vi "Weighted_Cross_Moments_1.vi"(0 "Cluster 1":T2={"Colour"=0, "Inst type"=enum."Pitot-static tube", "Inst name"="Manometer voltage", "Symbol"="U", "Code name"="", "Extra Info"="U", "Inst Array"=enum."PWA", "Index"=0, "Voltage Index"=0, "Extra Titles"=[], "Extra Values"=[], "Eng Values"=[], "Time (ms)"=[], "TT / Voltage"=[], "U"=0.0, "u^2"=0.0, "u^3"=0.0, "u^4"=0.0, "Skew_u"=0.0, "Kurt_u"=0.0, "Sd Error in Mean"=0.0, "% u'/U"=0.0, "X"=0.0, "Y"=0.0, "Z"=0.0, "Spectra"={"First Name"="", "Second Name"="", "X axis name"="", "Y axis name"="", "X array"=[], "Y array"=[]}, "Autocorrelation"={"First Name"="", "Second Name"="", "X axis name"="", "Y axis name"="", "X array"=[], "Y array"=[]}, "Timescale integral to 25%"=0.0, "Sd Error in Variance"=0.0, "Calib File"=path "", "Calib Constants"=[], "Histogram"={"First Name"="", "Second Name"="", "X axis name"="", "Y axis name"="", "X array"=[], "Y array"=[]}, "Output Position"=FALSE, "Full Stats"=FALSE} {"Sd Error in Variance" format="%.2f"; "Skew_u" format="%.2f"; "% u'/U" format="%.2f"; "Sd Error in Mean" format="%.2f"; "Kurt_u" format="%.2f"; "u^4" format="%.2f"; "u^3" format="%.2f"; "U" format="%.2f"; "u^2" format="%.2f"}, 1 "Cluster 2":T2={"Colour"=0, "Inst type"=enum."Pitot-static tube", "Inst name"="Manometer voltage", "Symbol"="U", "Code name"="", "Extra Info"="U", "Inst Array"=enum."PWA", "Index"=0, "Voltage Index"=0, "Extra Titles"=[], "Extra Values"=[], "Eng Values"=[], "Time (ms)"=[], "TT / Voltage"=[], "U"=0.0, "u^2"=0.0, "u^3"=0.0, "u^4"=0.0, "Skew_u"=0.0, "Kurt_u"=0.0, "Sd Error in Mean"=0.0, "% u'/U"=0.0, "X"=0.0, "Y"=0.0, "Z"=0.0, "Spectra"={"First Name"="", "Second Name"="", "X axis name"="", "Y axis name"="", "X array"=[], "Y array"=[]}, "Autocorrelation"={"First Name"="", "Second Name"="", "X axis name"="", "Y axis name"="", "X array"=[], "Y array"=[]}, "Timescale integral to 25%"=0.0, "Sd Error in Variance"=0.0, "Calib File"=path "", "Calib Constants"=[], "Histogram"={"First Name"="", "Second Name"="", "X axis name"="", "Y axis name"="", "X array"=[], "Y array"=[]}, "Output Position"=FALSE, "Full Stats"=FALSE} {"Sd Error in Variance" format="%.2f"; "Skew_u" format="%.2f"; "% u'/U" format="%.2f"; "Sd Error in Mean" format="%.2f"; "Kurt_u" format="%.2f"; "u^4" format="%.2f"; "u^3" format="%.2f"; "U" format="%.2f"; "u^2" format="%.2f"}, 5 "Shift in":dbl[](array[numeric]) format="%.2f") -> (17 "output cluster":T1 {"u^2w^2" format="%.2f"; "u^3w" format="%.2f"; "uw^3" format="%.2f"; "uw/u'w'" format="%.2f"; "uw^2" format="%.2f"; "u^2w" format="%.2f"; "uw" format="%.2f"}, 19 "Shift out":dbl[](array[numeric]) format="%.2f")   [LabVIEW 2011]
uses:
  Controls/Analysis_info_cluster.ctl
  Controls/Inst_type.ctl
  Controls/Instrument_Array.ctl
  Controls/XY_Plot_Cluster.ctl
  Controls/Correlation_cluster1.ctl
  Globals/Meas_global.vi
panel:
  in  "interp. method":i32(ring) items=["nearest", "linear", "spline", "cubic Hermite", "Lagrange"]
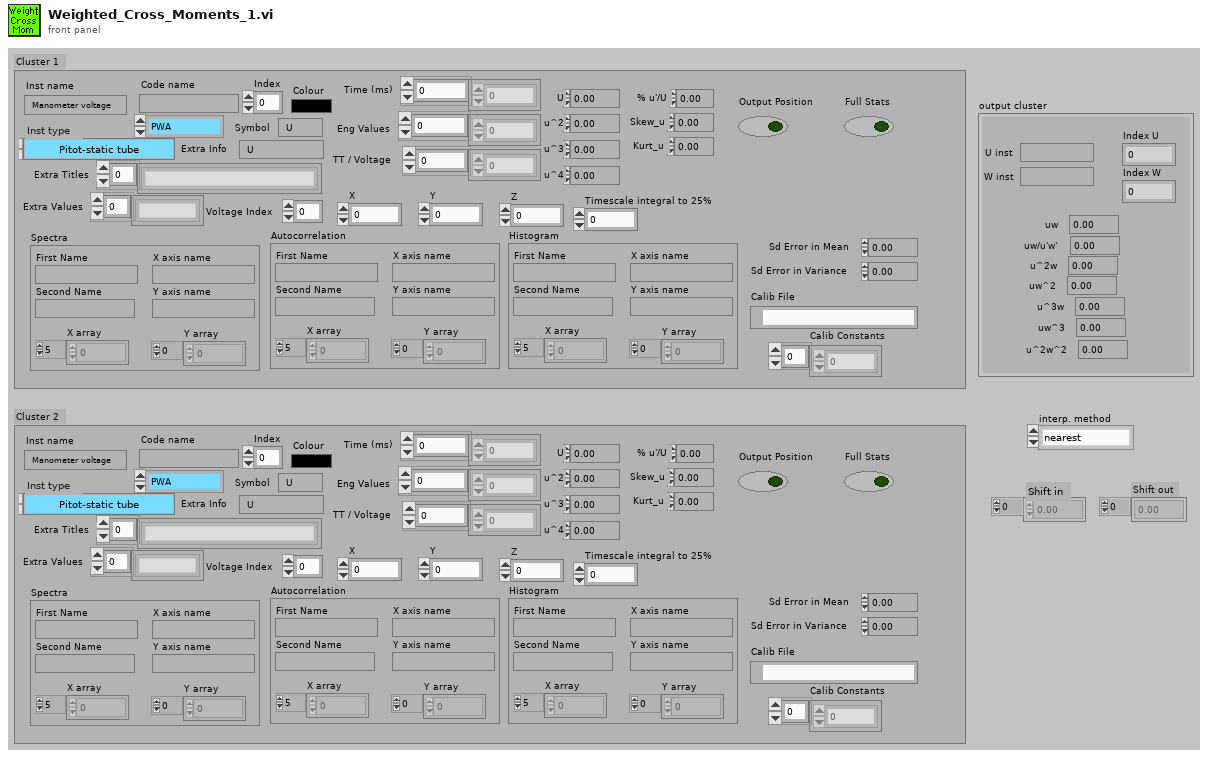
[diagram p1: front panel]
types:
  T1 = typedef "Correlation_cluster1.ctl" = cluster{"U inst":string, "uw":dbl, "u^2w":dbl, "uw^2":dbl, "uw/u'w'":dbl, "W inst":string, "uw^3":dbl, "u^3w":dbl, "u^2w^2":dbl, "Index U":i32, "Index W":i32}
  T2 = typedef "Analysis_info_cluster.ctl" = cluster{"Colour":u32, "Inst type":T3, "Inst name":string, "Symbol":string, "Code name":string, "Extra Info":string, "Inst Array":T4, "Index":i32, "Voltage Index":i32, "Extra Titles":string[], "Extra Values":string[], "Eng Values":dbl[], "Time (ms)":dbl[], "TT / Voltage":dbl[], "U":dbl, "u^2":dbl, "u^3":dbl, "u^4":dbl, "Skew_u":dbl, "Kurt_u":dbl, "Sd Error in Mean":dbl, "% u'/U":dbl, "X":dbl, "Y":dbl, "Z":dbl, "Spectra":T5, "Autocorrelation":T5, "Timescale integral to 25%":dbl, "Sd Error in Variance":dbl, "Calib File":path, "Calib Constants":dbl[], "Histogram":T5, "Output Position":bool, "Full Stats":bool}
  T3 = typedef "Inst_type.ctl" = enum16{"Propeller anemometer", "Raw voltage", "Pressure Transducer", "Pitot-static tube", "Preston tube", "Hot wire", "Cross wire 1", "Cross wire 2", "Generic Linear", "Generic Polynomial", "Generic BackPoly", "Fast FID", "Thermocouple", "Cold wire", "Pulsed Wire", "LDA Vel", "LDA Tran time", "LDA Arr time"}
  T4 = typedef "Instrument_Array.ctl" = enum16{"PWA", "LDA", "Analogue"}
  T5 = typedef "XY_Plot_Cluster.ctl" = cluster{"First Name":string, "Second Name":string, "X axis name":string, "Y axis name":string, "X array":dbl[], "Y array":dbl[]}
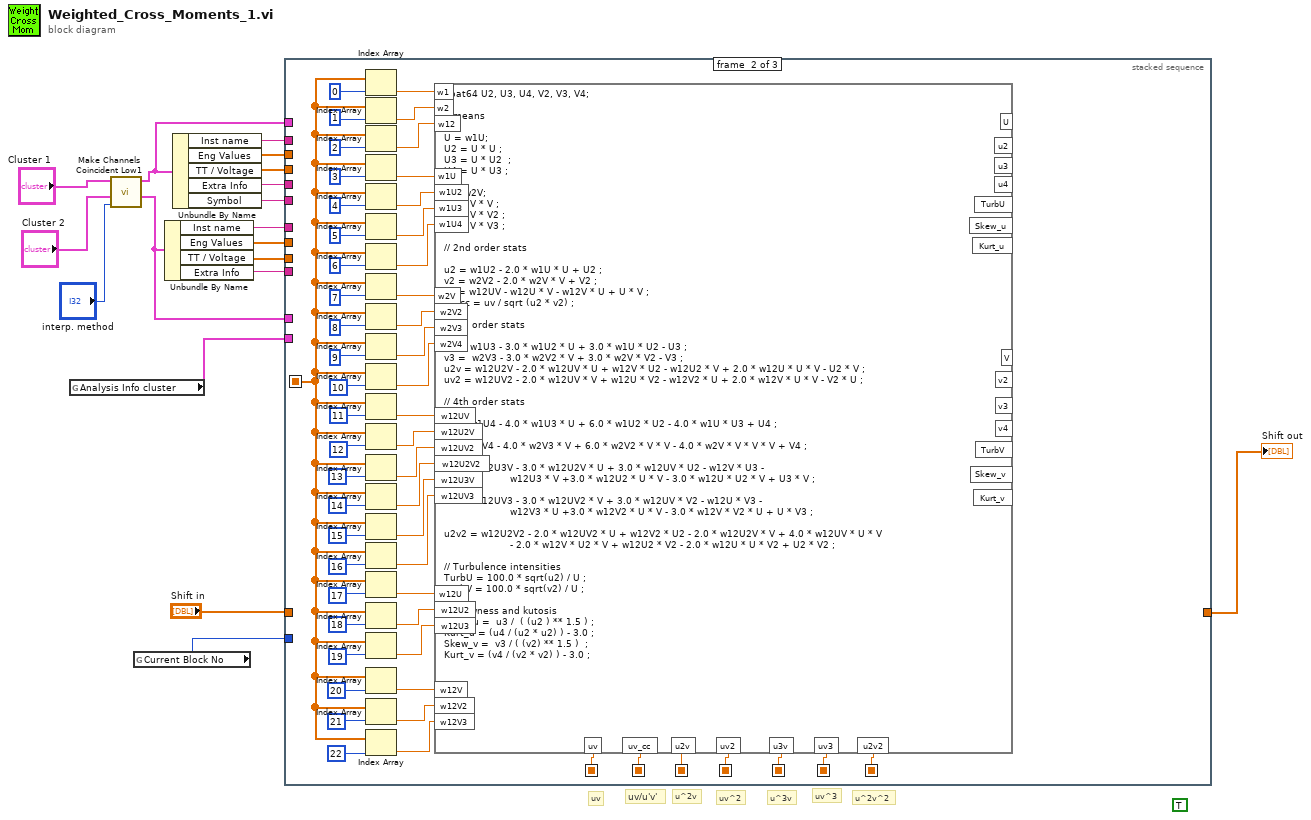
[diagram p0: block diagram]
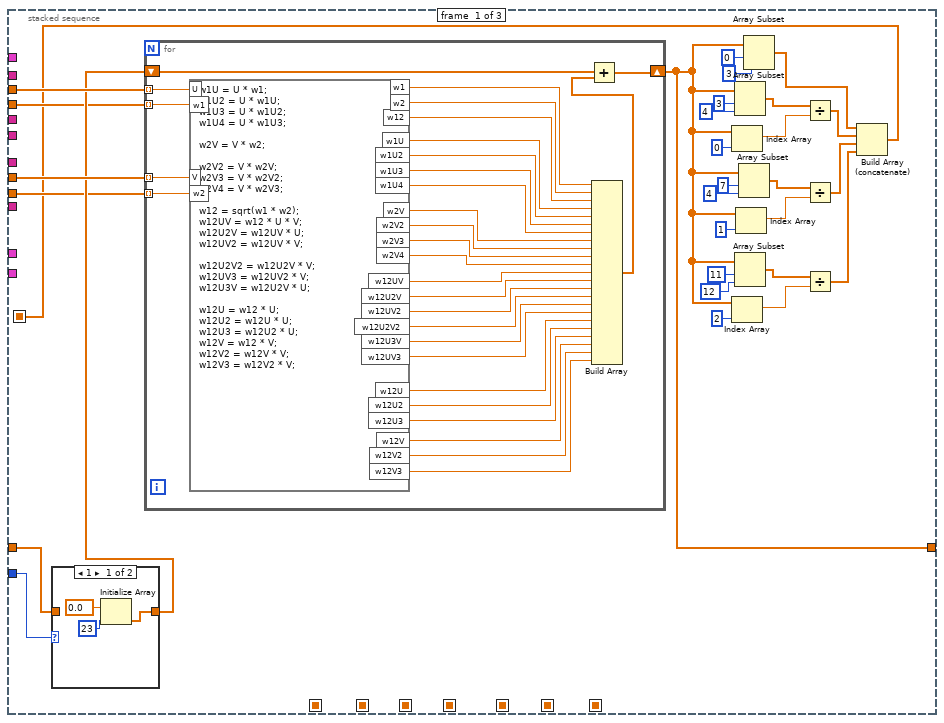
[diagram p2: hidden frame]
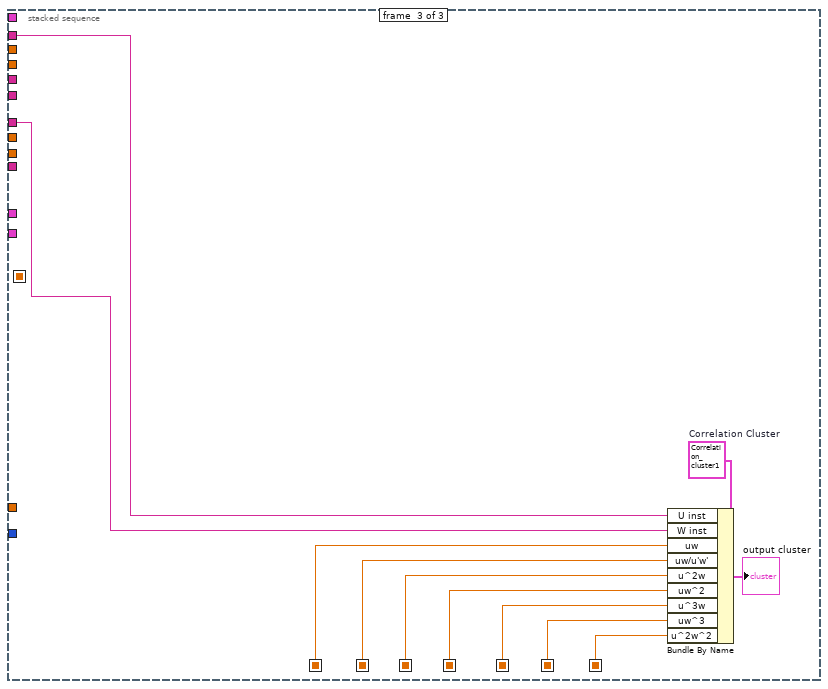
[diagram p4: hidden frame]
diagram:
  (unwired) TRUE
  # "u^2v^2"
  # "uv^3"
  # "u^3v"
  # "uv^2"
  # "u^2v"
  # "uv/u'v'"
  # "uv"
  n1 = global read "Meas_global.vi" "Analysis Info cluster"() -> (w14:T2[])
  n2 = call "Make Channels Coincident Low1.vi"("interp. method"="interp. method", "Cluster 2"="Cluster 2", "Cluster 1"="Cluster 1") -> ("Coincident Channel 2"=w4:T2, "Coincident Channel 1"=w5:T2)  [unwired: 7 in]
  n3 = global read "Meas_global.vi" "Current Block No"() -> (w9:i32)
  n4 = Unbundle By Name(w4) -> ("Inst name"=w10:string, "Eng Values"=w16:dbl[], "TT / Voltage"=w17:dbl[], "Extra Info"=w13:string)
  n5 = Unbundle By Name(w5) -> ("Inst name"=w11:string, "Eng Values"=w15:dbl[], "TT / Voltage"=w18:dbl[], "Extra Info"=w12:string, "Symbol"=w6:string)
  n6 = stacked-sequence {
    seq-local: [_ w124 _] -> [_ _ w144]
    seq-local: [_ w123 _] -> [_ _ w143]
    seq-local: [w41 _ _] -> [_ w85 _]
    seq-local: [_ w118 _] -> [_ _ w142]
    seq-local: [_ w117 _] -> [_ _ w141]
    seq-local: [_ w98 _] -> [_ _ w140]
    seq-local: [_ w97 _] -> [_ _ w139]
    seq-local: [_ w96 _] -> [_ _ w138]
    tunnel: w15 -> [w48 _ _]
    tunnel: "Shift in" -> [w45 _ _]
    tunnel: w16 -> [w47 _ _]
    tunnel: w14 -> [_ _ _]
    tunnel: w9 -> [w46 _ _]
    tunnel: w18 -> [w43 _ _]
    tunnel: w17 -> [w42 _ _]
    tunnel: w13 -> [_ _ _]
    tunnel: w12 -> [_ _ _]
    tunnel: w11 -> [_ _ w146]
    tunnel: w10 -> [_ _ w145]
    tunnel: [w40 _ _] -> w8
    tunnel: w6 -> [_ _ _]
    tunnel: w5 -> [_ _ _]
    tunnel: w4 -> [_ _ _]
    frame #0 {
      n7 = case shown="1" w46 {
        tunnel: [w49 w52] -> w44
        tunnel: w45 -> [_ w52]
        frame 1 {
          n8 = Initialize Array(0.0 ("Element Data"), 23 ("Dimension Size")) -> (w49:dbl[])
        }
        frame 2, Default {
        }
      }
      n9 = for {
        shift-right: [w78] -> w40
        shift-left: w44 -> [w82]
        tunnel: w43 -> [w77] mode=indexing
        tunnel: w48 -> [w80] mode=indexing
        tunnel: w47 -> [w79] mode=indexing
        tunnel: w42 -> [w76] mode=indexing
        n10 = formula code="w1U = U * w1;\nw1U2 = U * w1U;\nw1U3 = U * w1U2;\nw1U4 = U * w1U3;\n\nw2V = V * w2;\n\nw2V2 = V * w2V;\nw2V3 = V * w2V2;\nw2V4 = V * w2V3;\n\nw12 = sqrt(w1 * w2);\nw12UV = w12 * U * V;\nw12U2V = w12UV * U;\nw12UV2 = w12UV * V;\n\nw12U2V2 = w12U2V * V;\nw12UV3 = w12UV2 * V;\nw12U3V = w12U2V * U;\n\nw12U = w12 * U;\nw12U2 = w12U * U;\nw12U3 = w12U2 * U;\nw12V = w12 * V;\nw12V2 = w12V * V;\nw12V3 = w12V2 * V;"("V"=w79, "U"=w80, "w1"=w77, "w2"=w76) -> ("w12UV"=w67:dbl, "w1U"=w75:dbl, "w2V"=w71:dbl, "w1U2"=w74:dbl, "w2V2"=w70:dbl, "w12U2V"=w66:dbl, "w12UV2"=w65:dbl, "w1U3"=w73:dbl, "w1U4"=w72:dbl, "w2V3"=w69:dbl, "w2V4"=w68:dbl, "w12U3V"=w63:dbl, "w12UV3"=w62:dbl, "w12U2V2"=w64:dbl, "w12U"=w58:dbl, "w12U2"=w57:dbl, "w12U3"=w56:dbl, "w12V"=w55:dbl, "w12V2"=w54:dbl, "w12V3"=w53:dbl, "w12"=w61:dbl, "w1"=w60:dbl, "w2"=w59:dbl)
        n11 = Build Array(w60, w59, w61, w75, w74, w73, w72, w71, w70, w69, w68, w67, w66, w65, w64, w63, w62, w58, w57, w56, w55, w54, w53) -> (w81:dbl[])
        n12 = Add(x=w82, y=w81) -> (x+y=w78:dbl[])
      }
      n13 = Index Array(array=w40, index=0 ("Index")) -> (element=w36:dbl)
      n14 = Index Array(array=w40, index=2 ("Index")) -> (element=w26:dbl)
      n15 = Array Subset(array=w40, index=3 ("Array Index"), length=4) -> (w37:dbl[])
      n16 = Array Subset(array=w40, index=11 ("Array Index"), length=12) -> (w27:dbl[])
      n17 = Index Array(array=w40, index=1 ("Index")) -> (element=w33:dbl)
      n18 = Array Subset(array=w40, index=7 ("Array Index"), length=4) -> (w32:dbl[])
      n19 = Array Subset(array=w40, index=0, length=3) -> (w19:dbl[])
      n20 = Divide(x=w37, y=w36) -> (x/y=w24:dbl[])
      n21 = Divide(x=w32, y=w33) -> (x/y=w23:dbl[])
      n22 = Divide(x=w27, y=w26) -> (x/y=w22:dbl[])
      n23 = Build Array (concatenate)(w19, w24, w23, w22) -> (w41:dbl[])
    }
    frame #1 {
      n24 = Index Array(array=w85, index=0) -> (element=w130:dbl)
      n25 = Index Array(array=w85, index=1) -> (element=w129:dbl)
      n26 = Index Array(array=w85, index=2) -> (element=w128:dbl)
      n27 = Index Array(array=w85, index=3) -> (element=w127:dbl)
      n28 = Index Array(array=w85, index=4) -> (element=w126:dbl)
      n29 = Index Array(array=w85, index=5) -> (element=w125:dbl)
      n30 = Index Array(array=w85, index=6) -> (element=w120:dbl)
      n31 = Index Array(array=w85, index=7) -> (element=w119:dbl)
      n32 = Index Array(array=w85, index=8) -> (element=w110:dbl)
      n33 = Index Array(array=w85, index=9) -> (element=w109:dbl)
      n34 = Index Array(array=w85, index=10) -> (element=w112:dbl)
      n35 = Index Array(array=w85, index=11) -> (element=w111:dbl)
      n36 = Index Array(array=w85, index=12) -> (element=w106:dbl)
      n37 = Index Array(array=w85, index=13) -> (element=w105:dbl)
      n38 = Index Array(array=w85, index=14) -> (element=w101:dbl)
      n39 = Index Array(array=w85, index=15) -> (element=w100:dbl)
      n40 = Index Array(array=w85, index=16) -> (element=w99:dbl)
      n41 = Index Array(array=w85, index=17) -> (element=w91:dbl)
      n42 = Index Array(array=w85, index=18) -> (element=w90:dbl)
      n43 = Index Array(array=w85, index=19) -> (element=w89:dbl)
      n44 = Index Array(array=w85, index=20) -> (element=w88:dbl)
      n45 = Index Array(array=w85, index=21) -> (element=w84:dbl)
      n46 = Index Array(array=w85, index=22) -> (element=w83:dbl)
      n47 = formula code="float64 U2, U3, U4, V2, V3, V4;\n\n// means\n\nU = w1U;\nU2 = U * U ;\nU3 = U * U2  ;\nU4 = U * U3 ;\n\nV = w2V;\nV2 = V * V ;\nV3 = V * V2 ;\nV4 = V * V3 ;\n\n// 2nd order stats\n\nu2 = w1U2 - 2.0 * w1U * U + U2 ;\nv2 = w2V2 - 2.0 * w2V * V + V2 ;\nuv = w12UV - w12U * V - w12V * U + U * V ;\nuv_cc = uv / sqrt (u2 * v2) ;\n\n// 3rd order stats\n\nu3 = w1U3 - 3.0 * w1U2 * U + 3.0 * w1U * U2 - U3 ;\nv3 =  w2V3 - 3.0 * w2V2 * V + 3.0 * w2V * V2 - V3 ;\nu2v = w12U2V - 2.0 * w12UV * U + w12V * U2 - w12U2 * V + 2.0 * w12U * U * V - U2 * V ;\nuv2 = w12UV2 - 2.0 * w12UV * V + w12U * V2 - w12V2 * U + 2.0 * w12V * U * V - V2 * U ;\n\n// 4th order stats\n\nu4 = w1U4 - 4.0 * w1U3 * U + 6.0 * w1U2 * U2 - 4.0 * w1U * U3 + U4 ;\n\nv4 = w2V4 - 4.0 * w2V3 * V + 6.0 * w2V2 * V * V - 4.0 * w2V * V * V * V + V4 ;\n\nu3v = w12U3V - 3.0 * w12U2V * U + 3.0 * w12UV * U2 - w12V * U3 - \n                      w12U3 * V +3.0 * w12U2 * U * V - 3.0 * w12U * U2 * V + U3 * V ;\n\nuv3 = w12UV3 - 3.0 * w12UV2 * V + 3.0 * w12UV * V2 - w12U * V3 - \n                      w12V3 * U +3.0 * w12V2 * U * V - 3.0 * w12V * V2 * U + U * V3 ;\n\nu2v2 = w12U2V2 - 2.0 * w12UV2 * U + w12V2 * U2 - 2.0 * w12U2V * V + 4.0 * w12UV * U * V\n                      - 2.0 * w12V * U2 * V + w12U2 * V2 - 2.0 * w12U * U * V2 + U2 * V2 ; \n\n// Turbulence intensities\nTurbU = 100.0 * sqrt(u2) / U ;\nTurbV = 100.0 * sqrt(v2) / U ;\n\n// Skewness and kutosis\nSkew_u =  u3 /  ( (u2 ) ** 1.5 ) ;\nKurt_u = (u4 / (u2 * u2) ) - 3.0 ;\nSkew_v =  v3 / ( (v2) ** 1.5 )  ;\nKurt_v = (v4 / (v2 * v2) ) - 3.0 ;"("w1"=w130, "w2"=w129, "w12"=w128, "w1U2"=w126, "w1U3"=w125, "w1U"=w127, "w1U4"=w120, "w2V"=w119, "w2V2"=w110, "w2V4"=w112, "w2V3"=w109, "w12UV"=w111, "w12U2V"=w106, "w12UV2"=w105, "w12U2V2"=w101, "w12U3V"=w100, "w12UV3"=w99, "w12U2"=w90, "w12U3"=w89, "w12V"=w88, "w12V2"=w84, "w12U"=w91, "w12V3"=w83) -> ("uv"=w124:dbl, "uv_cc"=w123:dbl, "u2v"=w118:dbl, "uv2"=w117:dbl, "u3v"=w98:dbl, "uv3"=w97:dbl, "u2v2"=w96:dbl)  [unwired: 14 out]
    }
    frame #2 {
      w147 = T1 {"U inst"="", "uw"=0.0, "u^2w"=0.0, "uw^2"=0.0, "uw/u'w'"=0.0, "W inst"="", "uw^3"=0.0, "u^3w"=0.0, "u^2w^2"=0.0, "Index U"=0, "Index W"=0}  # Correlation Cluster
      n48 = Bundle By Name(cluster=w147, "U inst"=w146, "W inst"=w145, "uw"=w144, "uw/u'w'"=w143, "u^2w"=w142, "uw^2"=w141, "u^3w"=w140, "uw^3"=w139, "u^2w^2"=w138) -> (→"output cluster":T1)
    }
  }
  "Shift out" <- w8
